vi "TCP Connection Manager.vi"(6 "Properties In":T1, 8 "error in (no error)":errorcluster, 9 "Method":T4, 10 "Index":i32, 11 "Connection In":T2) -> (0 "error out":errorcluster, 1 "Number of Connections":i32, 2 "All Connections":T2[](array[typedef]), 3 "Connection Out":T2, 4 "Properties out":T1, 5 "All Properties":T1[](array[typedef]))   [LabVIEW 2014, in "QwaveSys Raspberry Pi Library.lvlib"]
doc: "This VI maintains the list of host connections."
uses:
  QwaveSys Raspberry Pi Library.lvlib
  stm_TCPConnectionMethod.ctl
  TCP/stm_TCP Connection Info.ctl
  _SubVIs/stm_MetaDataElement.ctl
  stm_TCPConnectionProperties.ctl
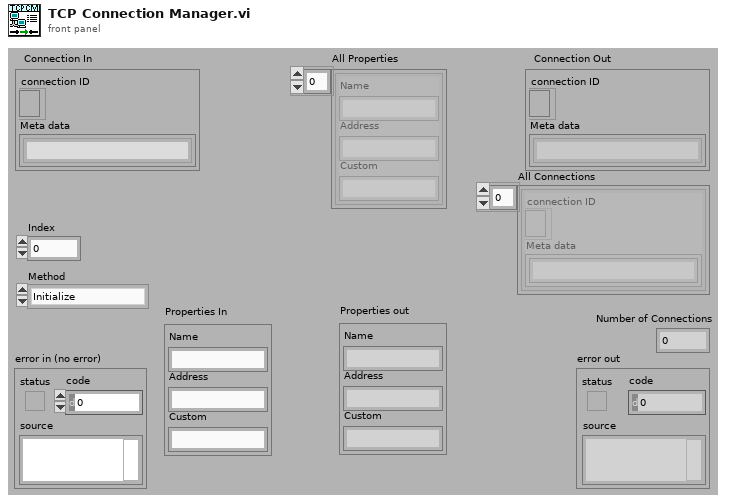
[diagram p1: front panel]
types:
  T1 = typedef "QwaveSys Raspberry Pi Library.lvlib/stm_TCPConnectionProperties.ctl" = cluster{"Name":string, "Address":string, "Custom":string}
  T2 = typedef "QwaveSys Raspberry Pi Library.lvlib/stm_TCP Connection Info.ctl" = cluster{"connection ID":refnum<k5>, "Meta data":T3[]}
  T3 = typedef "QwaveSys Raspberry Pi Library.lvlib/stm_MetaDataElement.ctl" = string
  T4 = typedef "QwaveSys Raspberry Pi Library.lvlib/stm_TCPConnectionMethod.ctl" = enum16{"Initialize", "Add Connection", "Set Properties", "Get Connection(s)", "Remove Connection", "Remove All Connections", "Get Connection Count"}
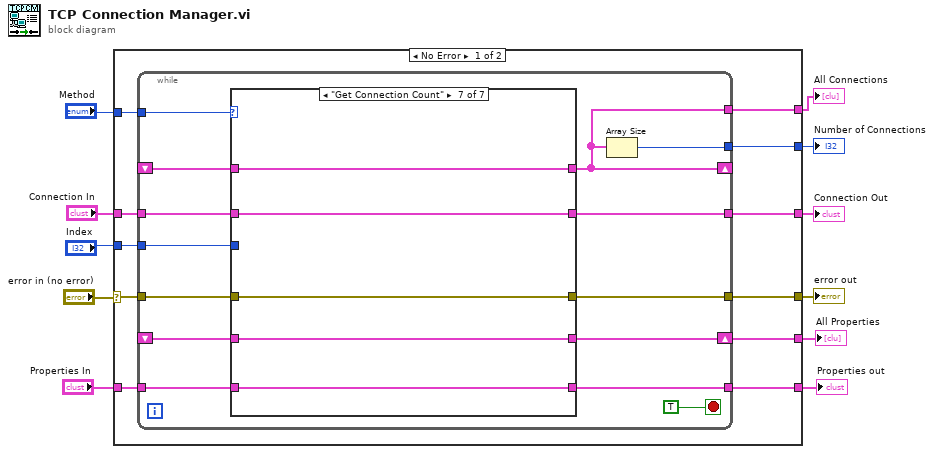
[diagram p0: block diagram]
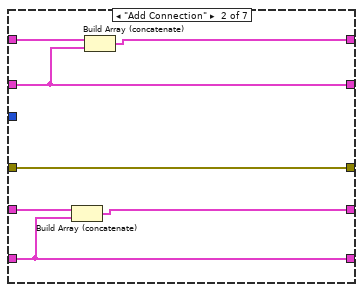
[diagram p3: hidden frame]
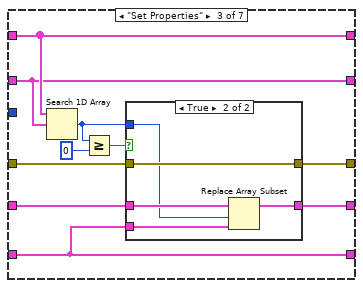
[diagram p4: hidden frame]
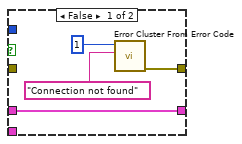
[diagram p5: hidden frame]
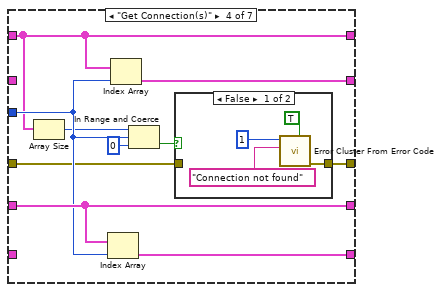
[diagram p6: hidden frame]
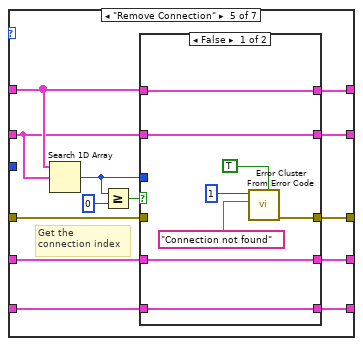
[diagram p8: hidden frame]
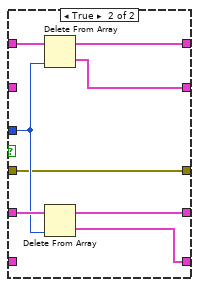
[diagram p9: hidden frame]
diagram:
  n1 = case shown="No Error" "error in (no error)" {
    selector: "error in (no error)" -> [w22 w115]
    tunnel: [w21 w115] -> w10
    tunnel: "Index" -> [w20 _]
    tunnel: "Method" -> [w19 _]
    tunnel: "Connection In" -> [w18 w114]
    tunnel: [w17 _] -> w6
    tunnel: [w16 _] -> w5
    tunnel: [w15 w114] -> w4
    tunnel: "Properties In" -> [w14 _]
    tunnel: [w13 _] -> w2
    tunnel: [w12 _] -> w1
    frame No Error {
      n2 = while {
        shift-right: [w28] -> _
        shift-left: _ -> [w35]
        tunnel: w22 -> [w34]
        tunnel: [w33] -> w21
        tunnel: w20 -> [w32]
        tunnel: w19 -> [w31]
        tunnel: w18 -> [w30]
        tunnel: [w29] -> w17
        tunnel: [w28] -> w16
        tunnel: [w27] -> w15
        shift-right: [w24] -> w13
        shift-left: _ -> [w26]
        tunnel: w14 -> [w25]
        tunnel: [w23] -> w12
        stop <- TRUE stop-if-true
        n3 = case shown="\"Get Connection Count\"" w31 {
          tunnel: w35 -> [_ w44 w53 w69 w91 _ w113]
          tunnel: w30 -> [_ w42 w52 _ w83 _ w112]
          tunnel: [_ w43 w53 w69 w87 _ w113] -> w28
          tunnel: [_ w42 w52 w73 w86 _ w112] -> w27
          tunnel: [w37 w41 w49 w64 w85 w108 w111] -> w33
          tunnel: w34 -> [w37 w41 w50 w67 w84 w108 w111]
          tunnel: w32 -> [_ _ _ w70 _ _ _]
          tunnel: w26 -> [_ w40 w48 w72 w82 _ w110]
          tunnel: w25 -> [_ w38 w45 _ w79 _ w109]
          tunnel: [_ w39 w46 w72 w81 _ w110] -> w24
          tunnel: [_ w38 w45 w71 w80 _ w109] -> w23
          frame "Initialize" {
          }
          frame "Add Connection" {
            n4 = Build Array (concatenate)(w40, w38) -> (w39:T1[])
            n5 = Build Array (concatenate)(w44, w42) -> (w43:T2[])
          }
          frame "Set Properties" {
            n6 = Search 1D Array(1D array=w53, element=w52) -> (index of element=w47:i32)  [unwired: 1 out]
            n7 = Greater Or Equal?(x=w47, y=0) -> (x >= y?=w51:bool)
            n8 = case shown="True" w51 {
              tunnel: w50 -> [_ w63]
              tunnel: [w55 w63] -> w49
              tunnel: w48 -> [w58 w62]
              tunnel: w47 -> [_ w61]
              tunnel: w45 -> [_ w60]
              tunnel: [w58 w59] -> w46
              frame False {
                n9 = call <vilib>:"Error Cluster From Error Code.vi"("error message (\"\")"="Connection not found" ("source"), "error code (0)"=1 ("code")) -> ("error out"=w55:errorcluster)  [unwired: 2 in, 5 out]
              }
              frame True {
                n10 = Replace Array Subset(array=w62, new element=w60, index=w61) -> (w59:T1[])
              }
            }
          }
          frame "Get Connection(s)" {
            n11 = Array Size(array=w69) -> (size(s)=w68:i32)
            n12 = Index Array(array=w72, index=w70) -> (element=w71:T1)
            n13 = Index Array(array=w69, index=w70) -> (element=w73:T2)
            n14 = In Range and Coerce(upper limit=w68, x=w70, lower limit=0) -> (In Range?=w66:bool)  [unwired: 1 out]
            n15 = case shown="False" w66 {
              tunnel: w67 -> [_ w78]
              tunnel: [w75 w78] -> w64
              frame False {
                n16 = call <vilib>:"Error Cluster From Error Code.vi"("is warning? (False)"=TRUE, "error message (\"\")"="Connection not found" ("source"), "error code (0)"=1 ("code")) -> ("error out"=w75:errorcluster)  [unwired: 2 in, 4 out]
              }
              frame True {
              }
            }
          }
          frame "Remove Connection" {
            # "Get the \nconnection index"
            n17 = Search 1D Array(1D array=w91, element=w83) -> (index of element=w90:i32)  [unwired: 1 out]
            n18 = Greater Or Equal?(x=w90, y=0) -> (x >= y?=w88:bool)
            n19 = case shown="False" w88 {
              tunnel: w91 -> [w99 w106]
              tunnel: w90 -> [_ w103]
              tunnel: [w99 w107] -> w87
              tunnel: [w98 w101] -> w86
              tunnel: [w95 w100] -> w85
              tunnel: w84 -> [_ w100]
              tunnel: w83 -> [w98 _]
              tunnel: w82 -> [w97 w105]
              tunnel: [w97 w104] -> w81
              tunnel: [w96 w102] -> w80
              tunnel: w79 -> [w96 _]
              frame False {
                n20 = call <vilib>:"Error Cluster From Error Code.vi"("is warning? (False)"=TRUE, "error message (\"\")"="Connection not found" ("source"), "error code (0)"=1 ("code")) -> ("error out"=w95:errorcluster)  [unwired: 2 in, 4 out]
              }
              frame True {
                n21 = Delete From Array(array=w106, index=w103) -> (deleted portion=w101:T2, array with subset deleted=w107:T2[])  [unwired: 1 in]
                n22 = Delete From Array(array=w105, index=w103) -> (deleted portion=w102:T1, array with subset deleted=w104:T1[])  [unwired: 1 in]
              }
            }
          }
          frame "Remove All Connections" {
          }
          frame "Get Connection Count" {
          }
        }
        n23 = Array Size(array=w28) -> (size(s)=w29:i32)
      }
    }
    frame Error {
    }
  }
  "error out" <- w10
  "Number of Connections" <- w6
  "All Connections" <- w5
  "Connection Out" <- w4
  "All Properties" <- w2
  "Properties out" <- w1
